vi "PathVelocityProfile.vi"(4 "DesAccel":dbl=15.0, 5 "intervalo":dbl=0.016, 6 "Accel":dbl=10.0, 7 "time":dbl, 8 "V_max":dbl format="%#_13g", 9 "Path  Smooth":dbl[][](array[numeric]), 10 "estimatives":T2, 11 "Pose":dbl[](array[numeric])) -> (2 "Vy":dbl, 3 "Vx":dbl)   [LabVIEW 2017]
uses:
  Controle/VelocityProfileState.ctl
  <vilib>/Analysis/coordinate.llb/Wrap Angle (scalar).vi
  <vilib>/Analysis/NI_AAL_Angle.lvlib
panel:
  in  "est_vy":dbl
  in  "est_vx":dbl
  out "VelocityProfile Y":T1[](array[typedef])
  out "VelocityProfile X":T1[](array[typedef])
  out "Velocity Profile Y":cluster{dbl[], dbl[]}[](graph)
  out "Velocity Profile X":cluster{dbl[], dbl[]}[](graph)
  out "Time Y":dbl[](array[numeric])
  out "Velocities Y":dbl[](array[numeric])
  out "Time X":dbl[](array[numeric])
  out "Velocities X":dbl[](array[numeric])
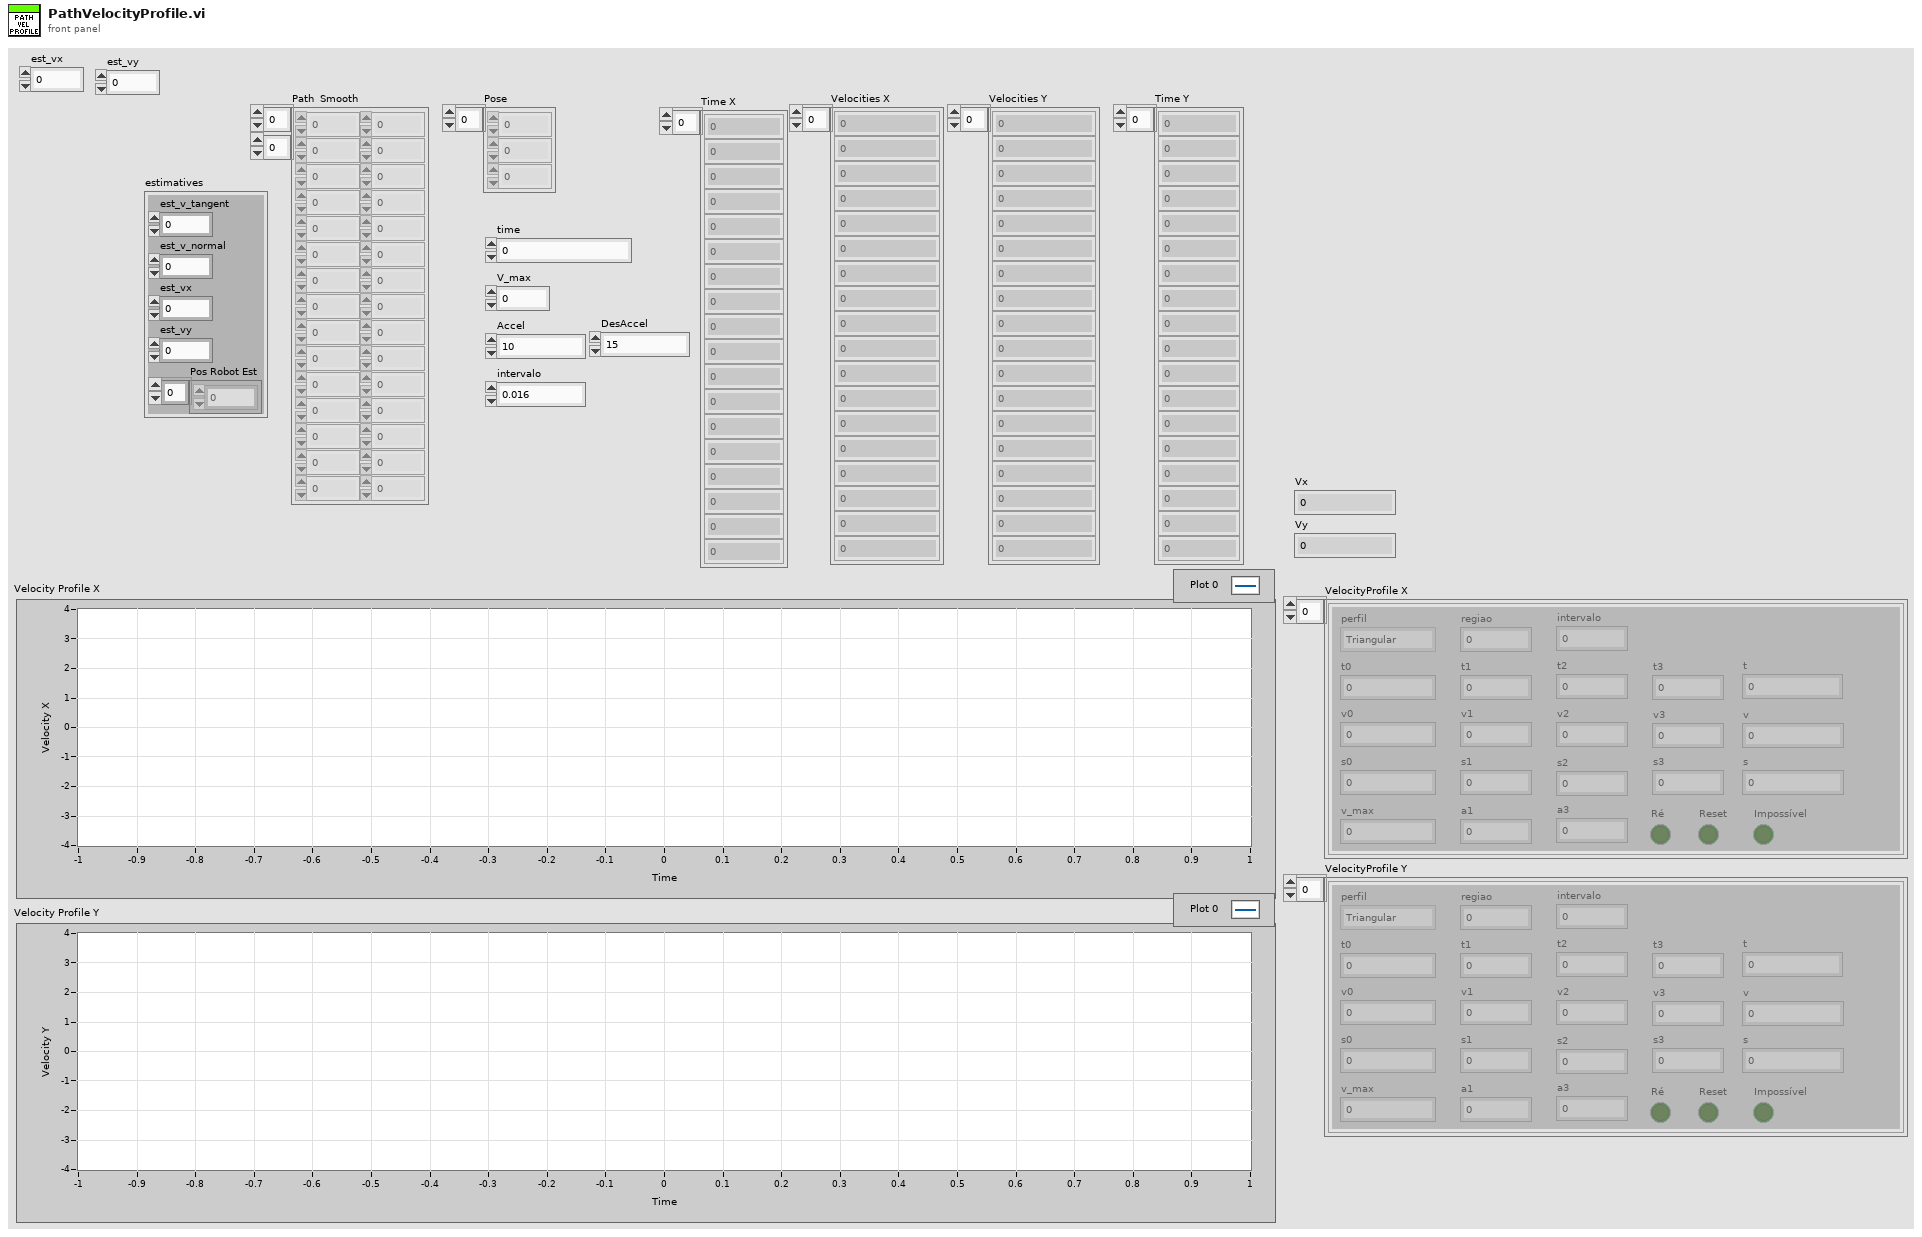
[diagram p1: front panel]
types:
  T1 = typedef "VelocityProfileState.ctl" = cluster{"t0":dbl, "t1":dbl, "t2":dbl, "t3":dbl, "v0":dbl, "v_max":dbl, "v3":dbl, "v2":dbl, "v1":dbl, "perfil":enum16{"Triangular", "Trapezoidal"}, "regiao":i32, "s0":dbl, "s1":dbl, "s2":dbl, "v":dbl, "t":dbl, "a1":dbl, "s3":dbl, "Reset":bool, "s":dbl, "a3":dbl, "Ré":bool, "Impossível":bool, "intervalo":dbl}
  T2 = cluster{"est_v_tangent":dbl, "est_v_normal":dbl, "est_vx":dbl, "est_vy":dbl, "Pos Robot Est":dbl[]}
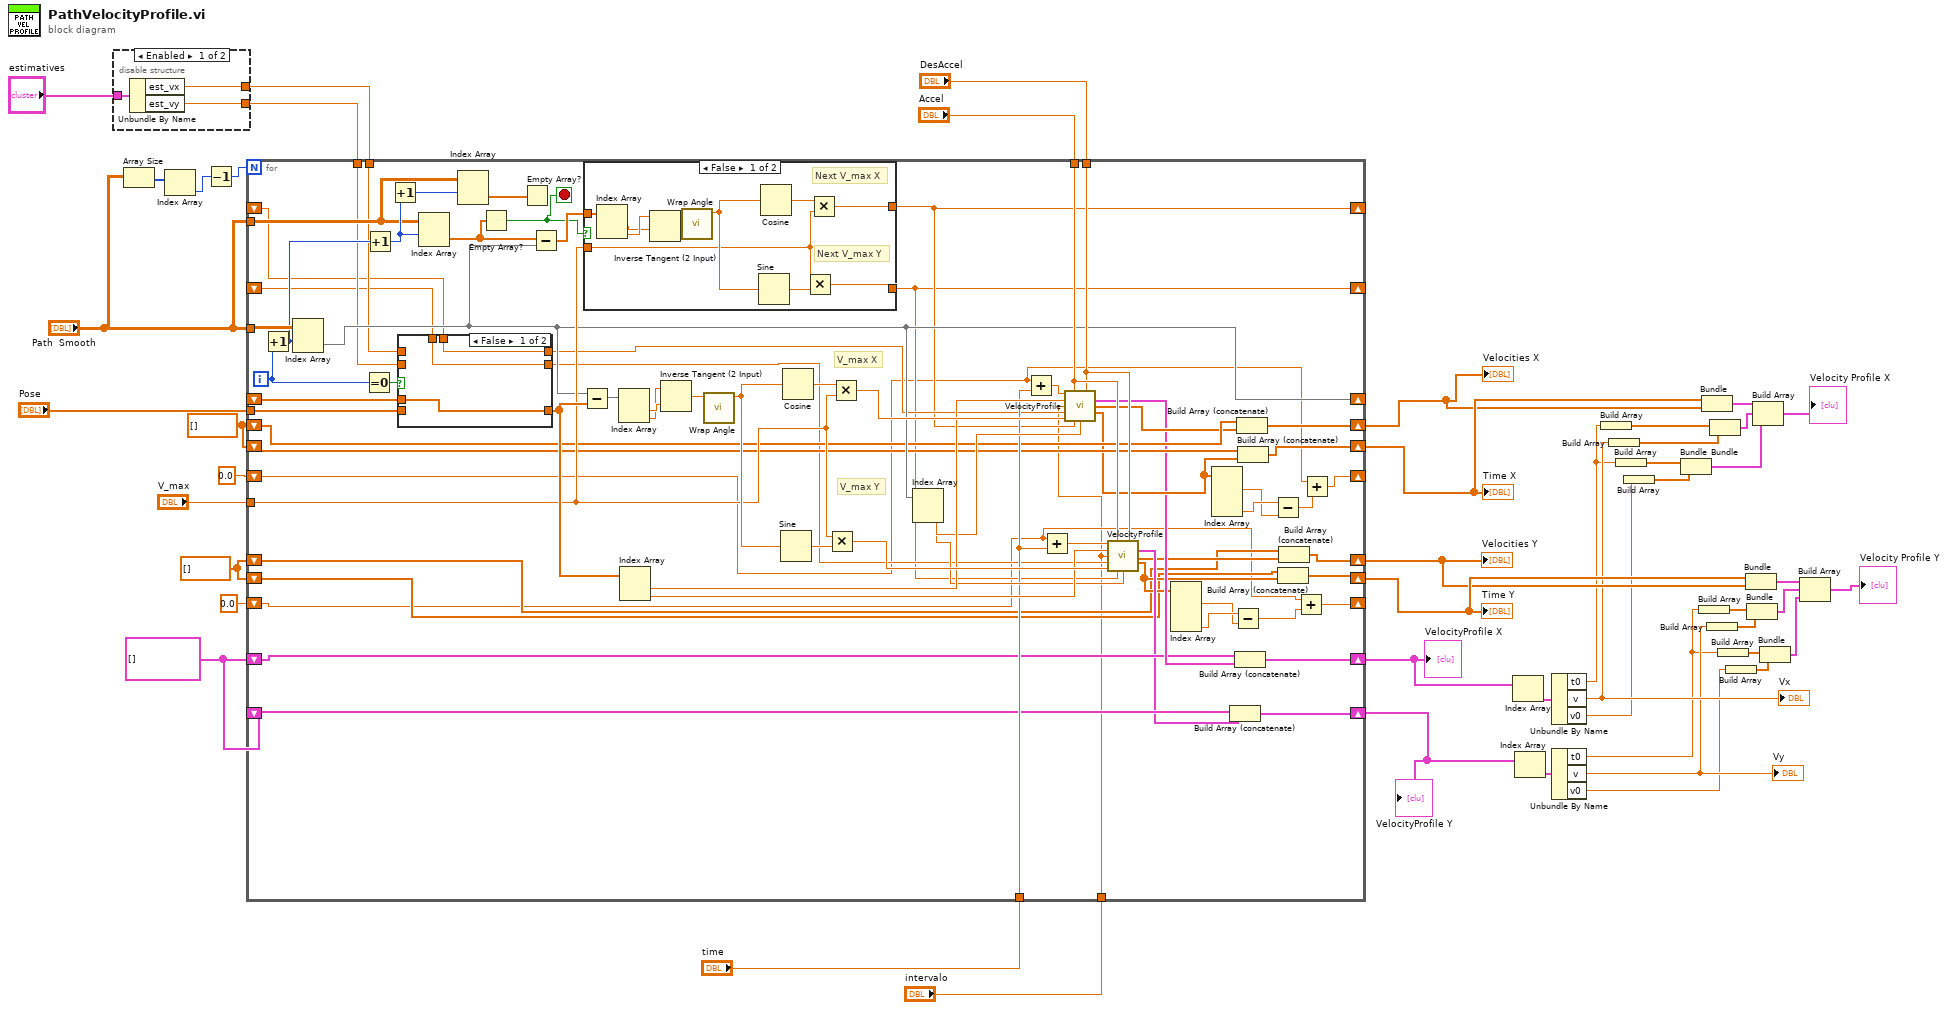
[diagram p0: block diagram]
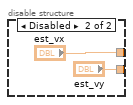
[diagram p2: hidden frame]
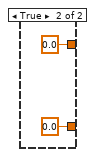
[diagram p3: hidden frame]
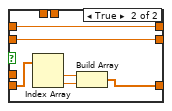
[diagram p4: hidden frame]
diagram:
  w28 = T1[] []
  w30 = dbl[] []
  w29 = dbl[] []
  n1 = disable-structure shown="Enabled" {
    disable-tunnel: "estimatives" -> [w51 _]
    disable-tunnel: [w50 "est_vx"] -> w32
    disable-tunnel: [w49 "est_vy"] -> w31
    frame Enabled {
      n2 = Unbundle By Name(w51) -> ("est_vx"=w50:dbl, "est_vy"=w49:dbl)
    }
    frame Disabled {
    }
  }
  n3 = Array Size(array="Path  Smooth") -> (size(s)=w39:i32[])
  n4 = Index Array(array=w39) -> (element=w38:i32)  [unwired: 1 in]
  n5 = Decrement(x=w38) -> (x-1=w37:i32)
  n6 = for {
    N: w37 -> [_]
    tunnel: "Path  Smooth" -> [w96]
    tunnel: "Pose" -> [w123]
    shift-right: [w97] -> _
    shift-left: _ -> [w122]
    tunnel: "V_max" -> [w103]
    tunnel: "Accel" -> [w113]
    tunnel: "DesAccel" -> [w112]
    tunnel: "Path  Smooth" -> [w106]
    shift-right: [w58] -> _
    shift-left: 0.0 ("t3") -> [w60]
    shift-right: [w56] -> _
    shift-left: 0.0 ("t3") -> [w55]
    tunnel: "time" -> [w99]
    shift-right: [w87] -> w35
    shift-left: w29 -> [w92]
    shift-right: [w90] -> w36
    shift-left: w29 -> [w91]
    shift-right: [w64] -> w33
    shift-left: w30 -> [w62]
    shift-right: [w63] -> w34
    shift-left: w30 -> [w61]
    tunnel: w32 -> [w84]
    tunnel: w31 -> [w83]
    shift-right: [w80] -> _
    shift-left: _ -> [w78]
    shift-right: [w79] -> _
    shift-left: _ -> [w77]
    shift-right: [w69] -> w26
    shift-left: w28 -> [w72]
    shift-right: [w68] -> w25
    shift-left: w28 -> [w71]
    tunnel: "intervalo" -> [w54]
    i -> [w95]
    stop <- w85 stop-if-true
    # "V_max Y"
    # "V_max X"
    n7 = Increment(x=w95) -> (x+1=w89:i32)
    n8 = Index Array(array=w96, index (row)=w89) -> (element=w97:dbl[])  [unwired: 1 in]
    n9 = Equal To 0?(x=w95) -> (x = 0?=w124:bool)
    n10 = Increment(x=w89) -> (x+1=w107:i32)
    n11 = Increment(x=w107) -> (x+1=w105:i32)
    n12 = case shown="False" w124 {
      tunnel: w123 -> [_ w145]
      tunnel: [w139 w142] -> w114
      tunnel: w122 -> [w139 _]
      tunnel: w84 -> [_ w141]
      tunnel: w83 -> [_ w140]
      tunnel: [w137 w141] -> w82
      tunnel: [w138 w140] -> w81
      tunnel: w78 -> [w137 _]
      tunnel: w77 -> [w138 _]
      frame False {
      }
      frame True {
        n13 = Index Array(array=w145) -> (element #1=w144:dbl, element #2=w143:dbl)  [unwired: 2 in]
        n14 = Build Array(w144, w143) -> (w142:dbl[])
      }
    }
    n15 = Index Array(array=w106, index (row)=w107) -> (element=w93:dbl[])  [unwired: 1 in]
    n16 = Index Array(array=w106, index (row)=w105) -> (element=w94:dbl[])  [unwired: 1 in]
    n17 = Empty Array?(array=w93) -> (empty?=w85:bool)
    n18 = Empty Array?(array=w94) -> ()  [unwired: 1 out]
    n19 = Subtract(x=w93, y=w97) -> (x-y=w104:dbl[])
    n20 = Subtract(x=w97, y=w114) -> (x-y=w120:dbl[])
    n21 = case shown="False" w85 {
      tunnel: w104 -> [w129 _]
      tunnel: w103 -> [w127 _]
      tunnel: [w126 0.0] -> w80
      tunnel: [w125 0.0] -> w79
      frame False {
        # "Next V_max Y"
        # "Next V_max X"
        n22 = Index Array(array=w129) -> (element #1=w128:dbl, element #2=w130:dbl)  [unwired: 2 in]
        n23 = Inverse Tangent (2 Input)(1:w128, 2:w130) -> (0:w131:dbl)
        n24 = call-poly <vilib>:"Wrap Angle.vi"("angle in"=w131) -> ("angle out"=w132:dbl)  [unwired: 9 in, 1 out]
        n25 = Sine(x=w132) -> (sin(x)=w134:dbl)
        n26 = Cosine(x=w132) -> (cos(x)=w133:dbl)
        n27 = Multiply(x=w127, y=w134) -> (x*y=w125:dbl)
        n28 = Multiply(x=w133, y=w127) -> (x*y=w126:dbl)
      }
      frame True {
      }
    }
    n29 = Index Array(array=w120) -> (element #1=w121:dbl, element #2=w119:dbl)  [unwired: 2 in]
    n30 = Index Array(array=w114) -> (element #1=w109:dbl, element #2=w108:dbl)  [unwired: 2 in]
    n31 = Inverse Tangent (2 Input)(1:w121, 2:w119) -> (0:w118:dbl)
    n32 = call-poly <vilib>:"Wrap Angle.vi"("angle in"=w118) -> ("angle out"=w117:dbl)  [unwired: 9 in, 1 out]
    n33 = Sine(x=w117) -> (sin(x)=w115:dbl)
    n34 = Cosine(x=w117) -> (cos(x)=w116:dbl)
    n35 = Multiply(x=w103, y=w115) -> (x*y=w110:dbl)
    n36 = Multiply(x=w116, y=w103) -> (x*y=w111:dbl)
    n37 = Index Array(array=w97) -> (element #1=w102:dbl, element #2=w101:dbl)  [unwired: 2 in]
    n38 = Add(x=w60, y=w99) -> (x+y=w100:dbl)
    n39 = Add(x=w55, y=w99) -> (x+y=w98:dbl)
    n40 = call "VelocityProfile.vi"("t"=w100, "a1"=w113, "a3"=w112, "s"=w109, "intervalo"=w54, "v_est"=w82, "v_max"=w111, "v3"=w80, "s3"=w102) -> ("VelocityProfileState Out"=w73:T1, "Velocities"=w88:dbl[], "Time"=w86:dbl[])  [unwired: 3 in, 1 out]
    n41 = call "VelocityProfile.vi"("t"=w98, "a1"=w113, "a3"=w112, "s"=w108, "intervalo"=w54, "v_est"=w81, "v_max"=w110, "v3"=w79, "s3"=w101) -> ("VelocityProfileState Out"=w70:T1, "Velocities"=w67:dbl[], "Time"=w65:dbl[])  [unwired: 3 in, 1 out]
    n42 = Index Array(array=w65) -> (element #1=w75:dbl, element #4=w76:dbl)  [unwired: 4 in, 2 out]
    n43 = Index Array(array=w86) -> (element #1=w66:dbl, element #4=w74:dbl)  [unwired: 4 in, 2 out]
    n44 = Build Array (concatenate)(w71, w70) -> (w68:T1[])
    n45 = Subtract(x=w76, y=w75) -> (x-y=w57:dbl)
    n46 = Build Array (concatenate)(w72, w73) -> (w69:T1[])
    n47 = Build Array (concatenate)(w92, w88) -> (w87:dbl[])
    n48 = Build Array (concatenate)(w91, w86) -> (w90:dbl[])
    n49 = Subtract(x=w74, y=w66) -> (x-y=w59:dbl)
    n50 = Build Array (concatenate)(w61, w65) -> (w63:dbl[])
    n51 = Build Array (concatenate)(w62, w67) -> (w64:dbl[])
    n52 = Add(x=w55, y=w57) -> (x+y=w56:dbl)
    n53 = Add(x=w60, y=w59) -> (x+y=w58:dbl)
  }
  "Velocities X" <- w35
  "Time X" <- w36
  "Velocities Y" <- w33
  "Time Y" <- w34
  "VelocityProfile X" <- w26
  "VelocityProfile Y" <- w25
  n54 = Index Array(array=w26) -> (element=w24:T1)  [unwired: 1 in]
  n55 = Index Array(array=w25) -> (element=w23:T1)  [unwired: 1 in]
  n56 = Unbundle By Name(w24) -> ("t0"=w8:dbl, "v"=w22:dbl, "v0"=w7:dbl)
  "Vx" <- w22
  n57 = Unbundle By Name(w23) -> ("t0"=w2:dbl, "v"=w14:dbl, "v0"=w1:dbl)
  "Vy" <- w14
  n58 = Build Array(w8) -> (w21:dbl[])
  n59 = Build Array(w22) -> (w20:dbl[])
  n60 = Build Array(w8) -> (w9:dbl[])
  n61 = Build Array(w7) -> (w10:dbl[])
  n62 = Bundle(w9, w10) -> (w6:cluster{dbl[], dbl[]})  [unwired: 1 in]
  n63 = Build Array(w2) -> (w15:dbl[])
  n64 = Bundle(w36, w35) -> (w19:cluster{dbl[], dbl[]})  [unwired: 1 in]
  n65 = Build Array(w14) -> (w16:dbl[])
  n66 = Bundle(w21, w20) -> (w18:cluster{dbl[], dbl[]})  [unwired: 1 in]
  n67 = Build Array(w2) -> (w3:dbl[])
  n68 = Build Array(w1) -> (w5:dbl[])
  n69 = Bundle(w34, w33) -> (w13:cluster{dbl[], dbl[]})  [unwired: 1 in]
  n70 = Bundle(w15, w16) -> (w12:cluster{dbl[], dbl[]})  [unwired: 1 in]
  n71 = Build Array(w19, w18, w6) -> (→"Velocity Profile X":cluster{dbl[], dbl[]}[])
  n72 = Bundle(w3, w5) -> (w4:cluster{dbl[], dbl[]})  [unwired: 1 in]
  n73 = Build Array(w13, w12, w4) -> (→"Velocity Profile Y":cluster{dbl[], dbl[]}[])
